vi "ReadAllDataByLabVIEW.vi"() -> ()   [LabVIEW 2020]
panel:
  in  "CreateSupportRequest":bool caption="Create\nSupport Request\n       Textfile"
  out "cSupportRequestText":string
  out "cProductModel":string caption="Product Model"
  out "cLastErrorPhase":string
  out "cLastErrorText":string
  out "clLastFWError":T1
  out "cModulesDisplay":string
  out "error out":errorcluster {"code" format="%9.0d"}
  out "iModuleCount":i32 caption="Modules"
  in  "error in (no error)":errorcluster
  out "cSerialNumber":string caption="Serial Number"
  in  "iDevIdx":i32 caption="Device Index" min=0 max=7 step=1
  in  "iPerformRestart":bool caption="Restart"
  out "cDescriptor":string caption="Descriptor"
  # "Module-by-Module\nSystem Analysis"
  # "System Description\nfor\nSupport Requests"
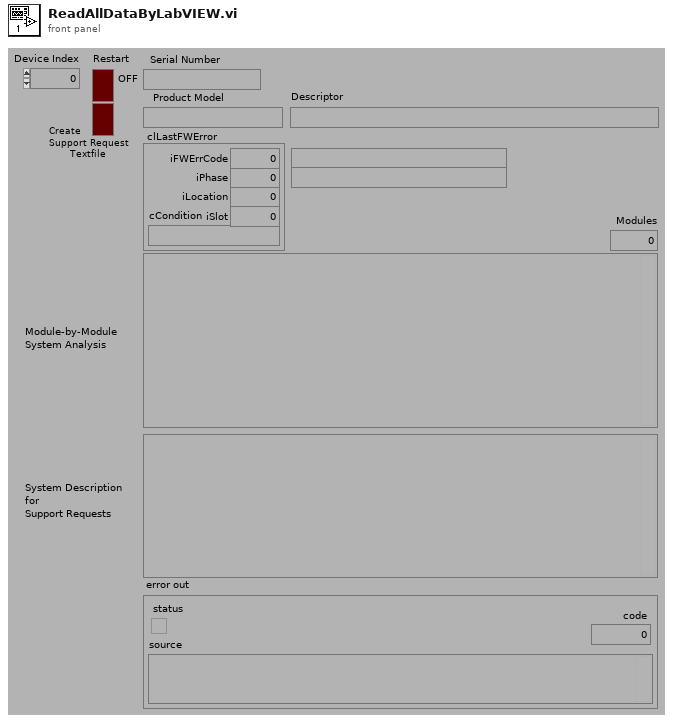
[diagram p1: front panel]
types:
  T1 = cluster{"iFWErrCode":i32, "iPhase":i32, "iLocation":i32, "iSlot":i32, "cCondition":string}
  T2 = cluster{"ErrCode":i32, "Error Text":string, "Phase":i32, "Phase Text":string, "Location":i32, "Slot":i32, "Condition":string}
  T3 = cluster{"SlotId":i32, "IsPrimary":u8, "IsBackPlane":u8, "HasUptimeCounter":u8}
  T4 = cluster{"TBNdxCount":u8, "MaxAmplitude":u16, "MaxSlewRate":u16, "ExpRampEffect":u16, "MinUserValue":u16, "MaxUserValue":u16, "UserResolution":u16}
  T5 = cluster{"TBNdx":u8, "PAPml":u16, "RRPml":u16, "PSPml":u16, "RSPml":u16, "WSPml":u16}
  T6 = cluster{"PumpState":enum8{"BOOST", "ECO"}, "PumpMode":enum8{"static", "dynamic"}}
  T7 = cluster{"Divider":u8, "PreSync":u8, "SyncMask":u8}
  T8 = cluster{"OutEnable":u8, "SyncEnable":u8, "SyncInverse":enum8{"Standard_Sync_Mask", "Inverse_Sync_Mask"}}
  T9 = cluster{"Divider":u16, "PreSync":u8, "SyncMask":u8}
  T10 = cluster{"Freq":i32, "PulseMode":u8, "HeadType":i32}
  T11 = cluster{"MainFreqTrig":string, "MainFreq":i32, "TrigLevelEnabled":u8}[]
  T12 = cluster{"MainFreqTrig":string, "MainFreq":i32, "TrigLevelEnabled":u8}
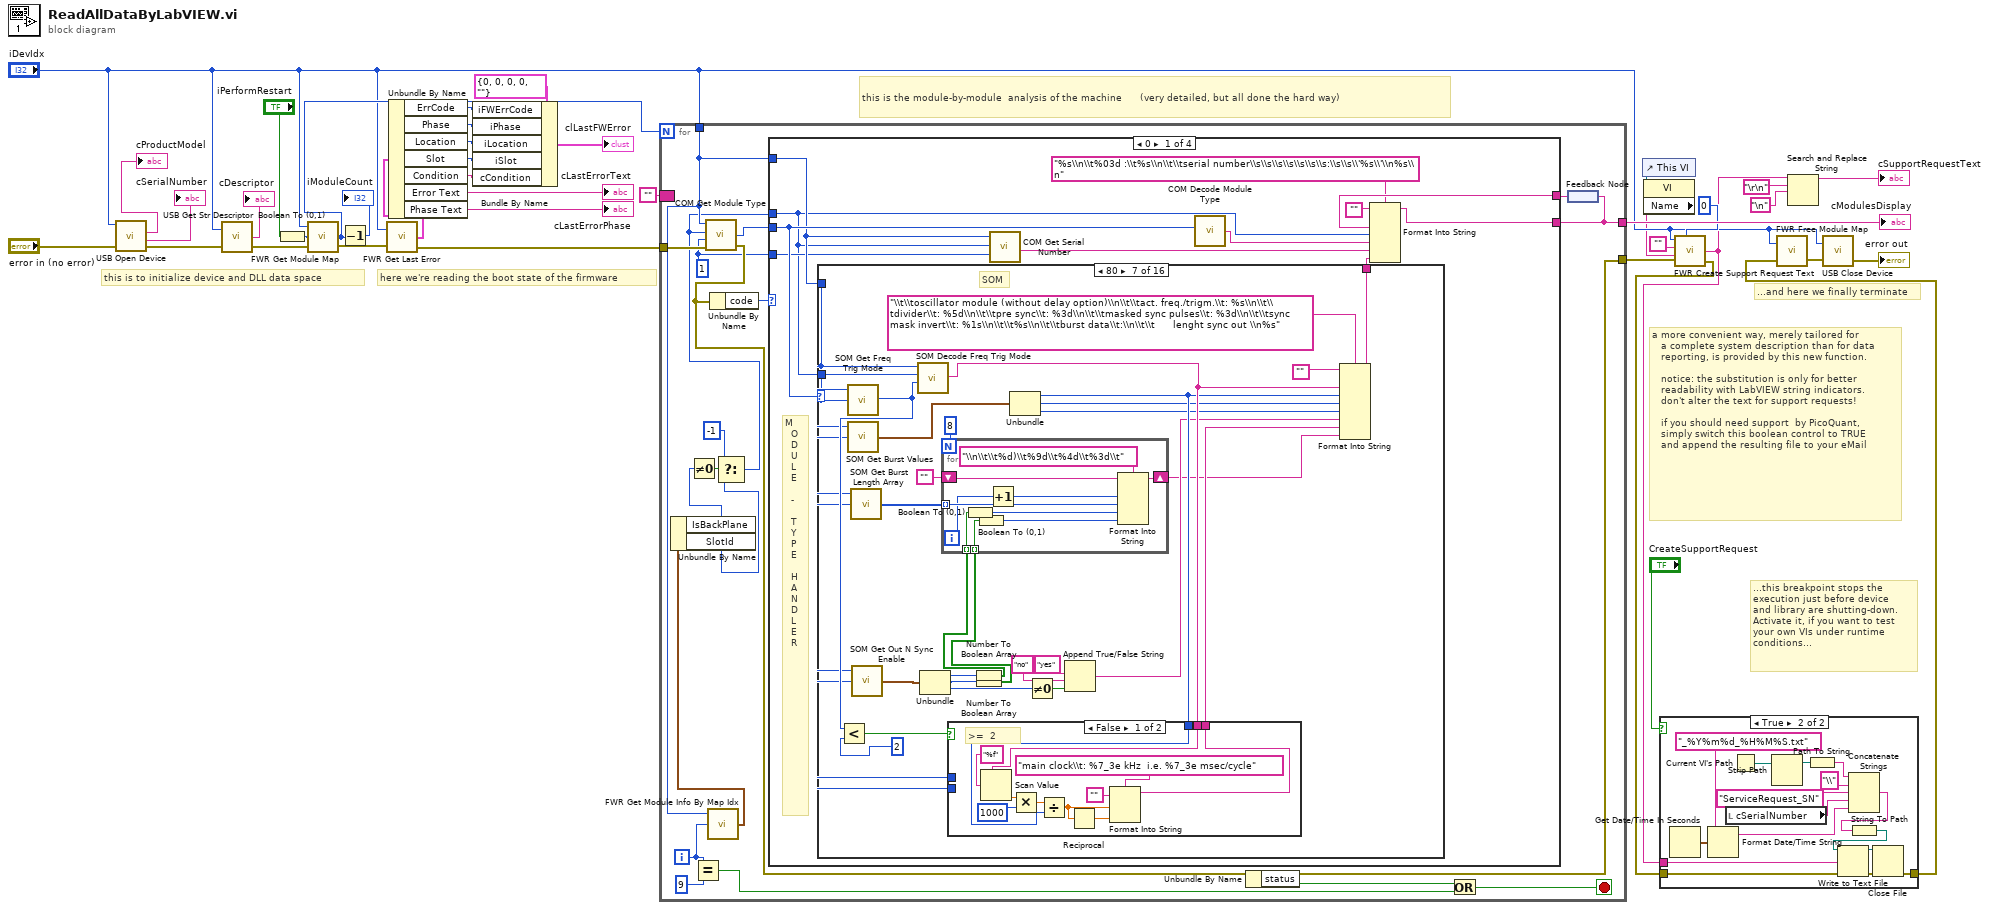
[diagram p0: block diagram]
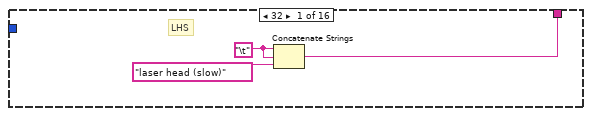
[diagram p3: hidden frame]
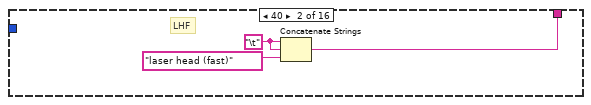
[diagram p4: hidden frame]
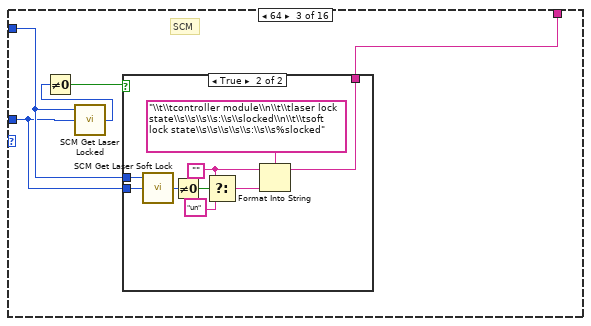
[diagram p5: hidden frame]
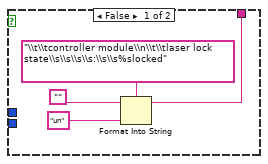
[diagram p6: hidden frame]
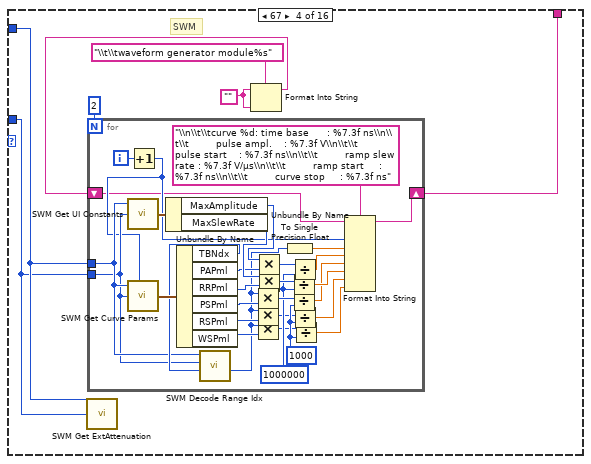
[diagram p7: hidden frame]
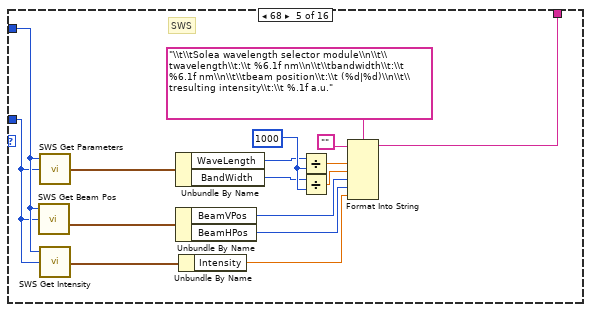
[diagram p8: hidden frame]
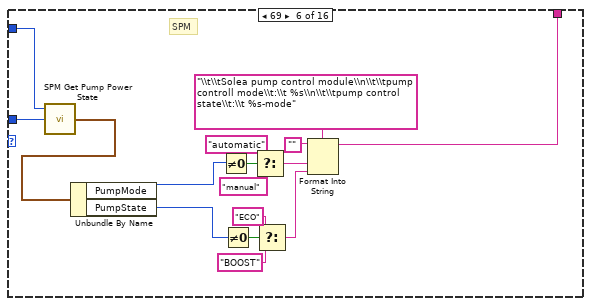
[diagram p9: hidden frame]
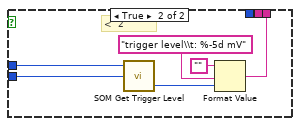
[diagram p10: hidden frame]
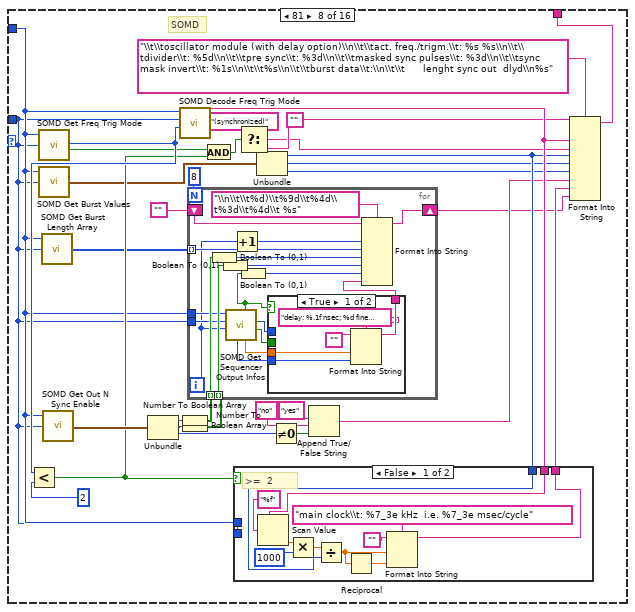
[diagram p11: hidden frame]
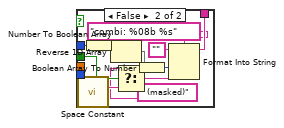
[diagram p12: hidden frame]
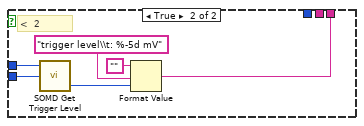
[diagram p13: hidden frame]
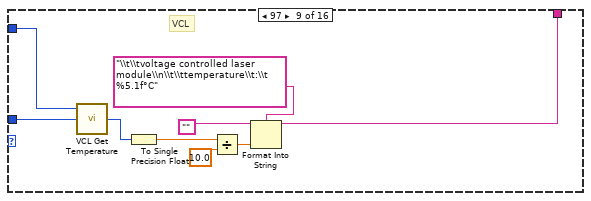
[diagram p14: hidden frame]
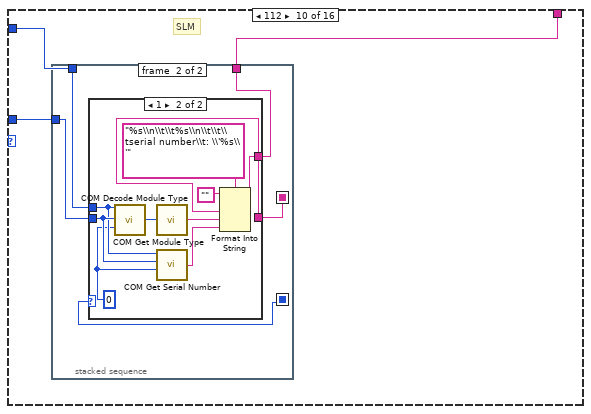
[diagram p15: hidden frame]
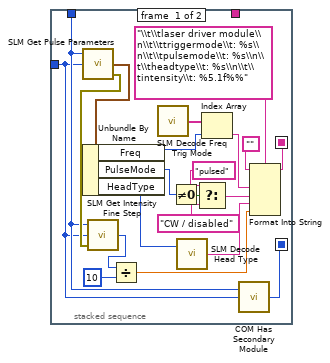
[diagram p16: hidden frame]
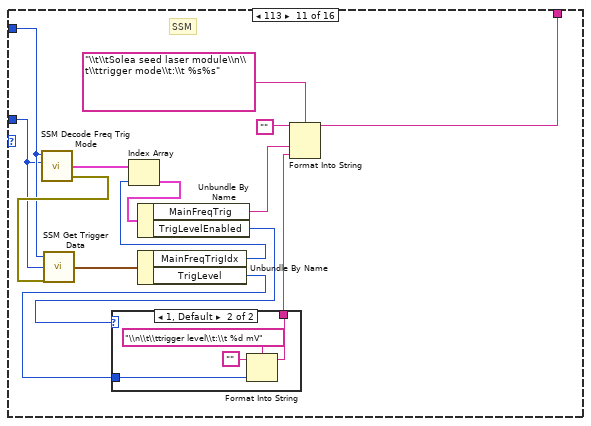
[diagram p18: hidden frame]
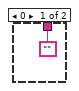
[diagram p19: hidden frame]
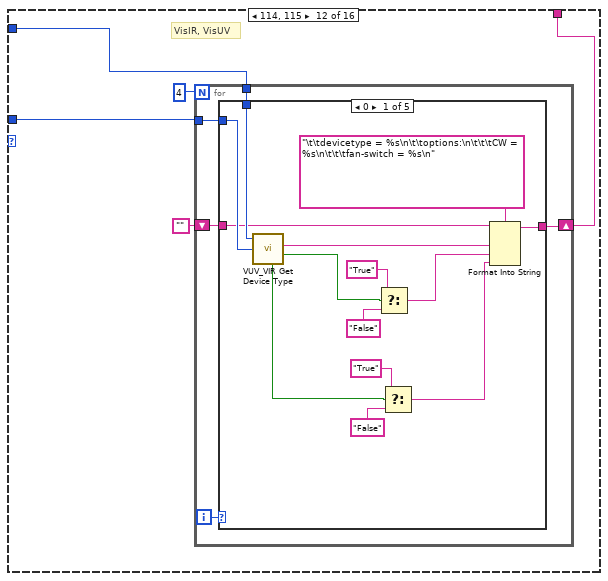
[diagram p20: hidden frame]
diagram:
  # "...this breakpoint stops the\nexecution just before device \nand library are shutting-down. \nActivate it, if you want to test \nyour own VIs under runtime \nconditions..."
  # "here we're reading the boot state of the firmware"
  # "a more convenient way, merely tailored for \n   a complete system description than for data      \n   reporting, is provided by this new function. \n\n   notice: the substitution is only for better  \n   readability with LabVIEW string indicators.\n   don't alter the text for support requests!\n\n   if you should need support  by PicoQuant,\n   simply switch this boolean control to TRUE\n   and append the resulting file to your eMail"
  # "...and here we finally terminate"
  # "this is the module-by-module  analysis of the machine      (very detailed, but all done the hard way)"
  # "this is to initialize device and DLL data space"
  n1 = call "USB Open Device.vi"("error in (no error)"="error in (no error)", "DevIdx"="iDevIdx") -> ("error out"=w36:errorcluster, "SerialNumber"=→"cSerialNumber":string, "ProductModel"=→"cProductModel":string)  [unwired: 2 in, 1 out]
  n2 = call "USB Get Str Descriptor.vi"("DevIdx"="iDevIdx", "error in (no error)"=w36) -> ("Descriptor"=→"cDescriptor":string, "error out"=w37:errorcluster)  [unwired: 1 out]
  n3 = Boolean To (0,1)(Boolean="iPerformRestart") -> (0, 1=w26:i16)
  n4 = call "FWR Get Module Map.vi"("error in (no error)"=w37, "PerformRestart"=w26, "DevIdx"="iDevIdx") -> ("error out"=w34:errorcluster, "ModuleCount"=w14:i32)  [unwired: 1 out]
  n5 = Decrement(x=w14) -> (x-1=→"iModuleCount":i32)
  n6 = call "FWR Get Last Error.vi"("DevIdx"="iDevIdx", "error in (no error)"=w34) -> ("Last Error"=w23:T2, "error out"=w33:errorcluster)  [unwired: 1 out]
  n7 = Unbundle By Name(w23) -> ("ErrCode"=w22:i32, "Phase"=w21:i32, "Location"=w20:i32, "Slot"=w19:i32, "Condition"=w18:string, "Error Text"=→"cLastErrorText":string, "Phase Text"=→"cLastErrorPhase":string)
  n8 = Bundle By Name(cluster=T1 {"iFWErrCode"=0, "iPhase"=0, "iLocation"=0, "iSlot"=0, "cCondition"=""} ("clLastFWError"), "iFWErrCode"=w22, "iPhase"=w21, "iLocation"=w20, "iSlot"=w19, "cCondition"=w18) -> (→"clLastFWError":T1)
  n9 = for {
    N: w14 -> [_]
    tunnel: "iDevIdx" -> [w45]
    tunnel: [w58] -> w29
    tunnel: w33 -> [w53]
    tunnel: [w52] -> w13
    border: "" -> [_]
    i -> [w48]
    stop <- w46 stop-if-true
    w50 = u8 1
    n10 = Equal?(x=w48, y=9) -> (x = y?=w55:bool)
    n11 = call "FWR Get Module Info By Map Idx.vi"("MapIdx"=w48, "DevIdx"=w45) -> ("FWR Module Info"=w47:T3)  [unwired: 1 in, 2 out]
    n12 = Unbundle By Name(w47) -> ("IsBackPlane"=w40:u8, "SlotId"=w42:i32)
    n13 = Not Equal To 0?(x=w40) -> (x != 0?=w44:bool)
    n14 = Select(t=-1, s=w44, f=w42) -> (s? t:f=w41:i32)
    n15 = call "COM Get Module Type.vi"("error in (no error)"=w53, "GetPrimary"=w50, "SlotId"=w41, "DevIdx"=w45) -> ("error out"=w52:errorcluster, "ModuleType"=w49:i32)  [unwired: 1 out]
    n16 = Unbundle By Name(w52) -> ("code"=w54:i32)
    n17 = Unbundle By Name(w52) -> ("status"=w51:bool)
    n18 = Or(x=w51, y=w55) -> (x .or. y?=w46:bool)
    n19 = feedback #1() -> (w57:string)
    n20 = case shown="0" w54 {
      tunnel: [w63 w604 w610 w616] -> w58
      tunnel: w57 -> [w65 w605 w611 w617]
      tunnel: w49 -> [w69 _ _ _]
      tunnel: w45 -> [w68 _ _ _]
      tunnel: w41 -> [w62 w603 w609 w615]
      tunnel: w50 -> [w67 _ _ _]
      frame 0 {
        # "M\n  O\n  D\n  U\n  L\n  E\n\n  -\n\n  T\n  Y\n  P\n  E\n\n  H\n  A\n  N\n  D\n  L\n  E\n  R"
        n21 = case shown="80" w69 {
          tunnel: [w70 w74 w76 w99 w133 w148 w190 w219 w303 w312 w352 w371 w446 w595 w598 "  oops?"] -> w59
          tunnel: w68 -> [_ _ w80 w98 w147 w163 w171 w221 w311 w314 w362 w375 w445 _ _ _]
          tunnel: w62 -> [_ _ w79 w97 w146 w162 w170 w220 w310 w313 w361 w374 w444 _ _ _]
          frame 32 {
            w72 = "\t"
            # "LHS"
            n22 = Concatenate Strings(w72, w72, "laser head (slow)") -> (w70:string)
          }
          frame 40 {
            w75 = "\t"
            # "LHF"
            n23 = Concatenate Strings(w75, w75, "laser head (fast)") -> (w74:string)
          }
          frame 64 {
            # "SCM"
            n24 = call "SCM Get Laser Locked.vi"("SlotId"=w79, "DevIdx"=w80) -> ("LaserLocked"=w78:enum8{"Laser unlocked", "Laser locked"})  [unwired: 1 in, 2 out]
            n25 = Not Equal To 0?(x=w78) -> (x != 0?=w77:bool)
            n26 = case shown="True" w77 {
              tunnel: [w82 w92] -> w76
              tunnel: w80 -> [_ w91]
              tunnel: w79 -> [_ w90]
              frame False {
                n27 = Format Into String(format string="\\t\\tcontroller module\\n\\t\\tlaser lock state\\s\\s\\s\\s:\\s\\s%slocked", initial string="", "un") -> (resulting string=w82:string)  [unwired: 1 in, 1 out]
              }
              frame True {
                w85 = ""
                n28 = call "SCM Get Laser Soft Lock.vi"("SlotId"=w90, "DevIdx"=w91) -> ("SoftLocked"=w87:enum8{"SoftLock off", "SoftLock on"})  [unwired: 1 in, 2 out]
                n29 = Not Equal To 0?(x=w87) -> (x != 0?=w86:bool)
                n30 = Select(t=w85, s=w86, f="un") -> (s? t:f=w89:string)
                n31 = Format Into String(format string="\\t\\tcontroller module\\n\\t\\tlaser lock state\\s\\s\\s\\s:\\s\\slocked\\n\\t\\tsoft lock state\\s\\s\\s\\s\\s:\\s\\s%slocked", initial string=w85, w89) -> (resulting string=w92:string)  [unwired: 1 in, 1 out]
              }
            }
          }
          frame 67 {
            w95 = ""
            # "SWM"
            n32 = call "SWM Get ExtAttenuation.vi"("SlotId"=w97, "DevIdx"=w98) -> ()  [unwired: 1 in, 3 out]
            n33 = Format Into String(format string="\\t\\twaveform generator module%s", initial string=w95, w95) -> (resulting string=w94:string)  [unwired: 1 in, 1 out]
            n34 = for {
              N: 2 -> [_]
              tunnel: w98 -> [w125]
              tunnel: w97 -> [w124]
              shift-right: [w116] -> w99
              shift-left: w94 -> [w115]
              i -> [w131]
              w110 = 1000
              w111 = 1000000
              n35 = call "SWM Get UI Constants.vi"("SlotId"=w124, "DevIdx"=w125) -> ("SWM UI Constants"=w123:T4)  [unwired: 1 in, 2 out]
              n36 = Increment(x=w131) -> (x+1=w118:i32)
              n37 = call "SWM Get Curve Params.vi"("DevIdx"=w125, "CurveIdx"=w118, "SlotId"=w124) -> ("SWM Curve Params"=w130:T5)  [unwired: 2 in, 2 out]
              n38 = Unbundle By Name(w123) -> ("MaxAmplitude"=w121:u16, "MaxSlewRate"=w122:u16)
              n39 = Unbundle By Name(w130) -> ("TBNdx"=w129:u8, "PAPml"=w120:u16, "RRPml"=w119:u16, "PSPml"=w128:u16, "RSPml"=w127:u16, "WSPml"=w126:u16)
              n40 = call "SWM Decode Range Idx.vi"("RangeIdx"=w129, "SlotId"=w124, "DevIdx"=w125) -> ("UpperLimit"=w101:i32)  [unwired: 2 in, 2 out]
              n41 = Multiply(x=w101, y=w128) -> (x*y=w112:u32)
              n42 = Multiply(x=w101, y=w127) -> (x*y=w109:u32)
              n43 = Multiply(x=w101, y=w126) -> (x*y=w108:u32)
              n44 = Multiply(x=w121, y=w120) -> (x*y=w114:u32)
              n45 = Multiply(x=w122, y=w119) -> (x*y=w113:u32)
              n46 = To Single Precision Float(number=w101) -> (single precision float=w102:sgl)
              n47 = Divide(x=w113, y=w111) -> (x/y=w105:sgl)
              n48 = Divide(x=w112, y=w110) -> (x/y=w104:sgl)
              n49 = Divide(x=w114, y=w111) -> (x/y=w103:sgl)
              n50 = Divide(x=w109, y=w110) -> (x/y=w106:sgl)
              n51 = Divide(x=w108, y=w110) -> (x/y=w107:sgl)
              n52 = Format Into String(format string="\\n\\t\\tcurve %d: time base      : %7.3f ns\\n\\t\\t         pulse ampl.    : %7.3f V\\n\\t\\t         pulse start    : %7.3f ns\\n\\t\\t         ramp slew rate : %7.3f V/µs\\n\\t\\t         ramp start     : %7.3f ns\\n\\t\\t         curve stop     : %7.3f ns", initial string=w115, w118, w102, w103, w104, w105, w106, w107) -> (resulting string=w116:string)  [unwired: 1 in, 1 out]
            }
          }
          frame 68 {
            w144 = 1000
            # "SWS"
            n53 = call "SWS Get Beam Pos.vi"("SlotId"=w146, "DevIdx"=w147) -> ("SWS Beam Pos"=w138:cluster{"BeamVPos":i16, "BeamHPos":i16})  [unwired: 1 in, 2 out]
            n54 = call "SWS Get Parameters.vi"("SlotId"=w146, "DevIdx"=w147) -> ("SWS Parameters"=w145:cluster{"WaveLength":u32, "BandWidth":u32})  [unwired: 1 in, 2 out]
            n55 = call "SWS Get Intensity.vi"("SlotId"=w146, "DevIdx"=w147) -> ("SWS Intensity"=w137:cluster{"IntensityRaw":u32, "Intensity":sgl})  [unwired: 1 in, 2 out]
            n56 = Unbundle By Name(w145) -> ("WaveLength"=w142:u32, "BandWidth"=w143:u32)
            n57 = Unbundle By Name(w138) -> ("BeamVPos"=w136:i16, "BeamHPos"=w135:i16)
            n58 = Unbundle By Name(w137) -> ("Intensity"=w134:sgl)
            n59 = Divide(x=w142, y=w144) -> (x/y=w140:sgl)
            n60 = Divide(x=w143, y=w144) -> (x/y=w139:sgl)
            n61 = Format Into String(format string="\\t\\tSolea wavelength selector module\\n\\t\\twavelength\\t:\\t %6.1f nm\\n\\t\\tbandwidth\\t:\\t %6.1f nm\\n\\t\\tbeam position\\t:\\t (%d|%d)\\n\\t\\tresulting intensity\\t:\\t %.1f a.u.", initial string="", w140, w139, w136, w135, w134) -> (resulting string=w133:string)  [unwired: 1 in, 1 out]
          }
          frame 69 {
            # "SPM"
            n62 = call "SPM Get Pump Power State.vi"("SlotId"=w162, "DevIdx"=w163) -> ("Pump Power State"=w161:T6)  [unwired: 1 in, 2 out]
            n63 = Unbundle By Name(w161) -> ("PumpMode"=w151:enum8{"static", "dynamic"}, "PumpState"=w150:enum8{"BOOST", "ECO"})
            n64 = Not Equal To 0?(x=w151) -> (x != 0?=w159:bool)
            n65 = Not Equal To 0?(x=w150) -> (x != 0?=w155:bool)
            n66 = Select(t="automatic", s=w159, f="manual") -> (s? t:f=w160:string)
            n67 = Select(t="ECO", s=w155, f="BOOST") -> (s? t:f=w152:string)
            n68 = Format Into String(format string="\\t\\tSolea pump control module\\n\\t\\tpump controll mode\\t:\\t %s\\n\\t\\tpump control state\\t:\\t %s-mode", initial string="", w160, w152) -> (resulting string=w148:string)  [unwired: 1 in, 1 out]
          }
          frame 80 {
            # "SOM"
            n69 = call "SOM Get Freq Trig Mode.vi"("SlotId"=w170, "DevIdx"=w171) -> ("FreqTrigMode"=w184:i32)  [unwired: 1 in, 2 out]
            n70 = Less?(x=w184, y=2) -> (x < y?=w183:bool)
            n71 = call "SOM Get Burst Values.vi"("SlotId"=w170, "DevIdx"=w171) -> ("SOM Burst Values"=w182:T7)  [unwired: 1 in, 2 out]
            n72 = call "SOM Get Burst Length Array.vi"("SlotId"=w170, "DevIdx"=w171) -> ("SOM Burst Length Array"=w180:i32[])  [unwired: 1 in, 2 out]
            n73 = call "SOM Get Out N Sync Enable.vi"("SlotId"=w170, "DevIdx"=w171) -> ("SOM Out N Sync Enable"=w187:T8)  [unwired: 1 in, 2 out]
            n74 = call "SOM Decode Freq Trig Mode.vi"("FreqTrigMode"=w184, "SlotId"=w170, "DevIdx"=w171) -> ("FreqTrigMode"=w188:string)  [unwired: 1 in, 2 out]
            n75 = Unbundle(w187) -> ("OutEnable"=w175:u8, "SyncEnable"=w176:u8, "SyncInverse"=w186:enum8{"Standard_Sync_Mask", "Inverse_Sync_Mask"})
            n76 = Number To Boolean Array(number=w175) -> (Boolean array=w174:bool[])
            n77 = Number To Boolean Array(number=w176) -> (Boolean array=w173:bool[])
            n78 = for {
              N: 8 -> [_]
              tunnel: w180 -> [w201] mode=indexing
              shift-right: [w198] -> w164
              shift-left: "" -> [w197]
              tunnel: w174 -> [w194] mode=indexing
              tunnel: w173 -> [w193] mode=indexing
              i -> [w192]
              n79 = Boolean To (0,1)(Boolean=w194) -> (0, 1=w196:i16)
              n80 = Boolean To (0,1)(Boolean=w193) -> (0, 1=w195:i16)
              n81 = Increment(x=w192) -> (x+1=w200:i32)
              n82 = Format Into String(format string="\\n\\t\\t%d)\\t%9d\\t%4d\\t%3d\\t", initial string=w197, w200, w201, w196, w195) -> (resulting string=w198:string)  [unwired: 1 in, 1 out]
            }
            n83 = Unbundle(w182) -> ("Divider"=w169:u8, "PreSync"=w168:u8, "SyncMask"=w167:u8)
            n84 = case shown="False" w183 {
              tunnel: w171 -> [_ w218]
              tunnel: w170 -> [_ w217]
              tunnel: [w211 w213] -> w165
              tunnel: w188 -> [w202 _]
              tunnel: w169 -> [w203 _]
              frame False {
                # ">=  2"
                n85 = Scan Value(string=w202, format string="%f") -> (value=w208:dbl)  [unwired: 1 in, 1 out]
                n86 = Multiply(x=w208, y=1000) -> (x*y=w206:dbl)
                n87 = Divide(x=w206, y=w203) -> (x/y=w205:dbl)
                n88 = Reciprocal(x=w205) -> (1/x=w204:dbl)
                n89 = Format Into String(format string="main clock\\t: %7_3e kHz  i.e. %7_3e msec/cycle", initial string="", w205, w204) -> (resulting string=w211:string)  [unwired: 1 in, 1 out]
              }
              frame True {
                # "<  2"
                n90 = call "SOM Get Trigger Level.vi"("SlotId"=w217, "DevIdx"=w218) -> ("MilliVolt"=w216:i32)  [unwired: 1 in, 2 out]
                n91 = Format Value(string ("")="", format string="trigger level\\t: %-5d mV", value (0)=w216) -> (output string=w213:string)
              }
            }
            n92 = Not Equal To 0?(x=w186) -> (x != 0?=w179:bool)
            n93 = Append True/False String(1:w179, 2:"no" ("false string"), 3:"yes" ("true string")) -> (0:w166:string)  [unwired: 1 in]
            n94 = Format Into String(format string="\\t\\toscillator module (without delay option)\\n\\t\\tact. freq./trigm.\\t: %s\\n\\t\\tdivider\\t: %5d\\n\\t\\tpre sync\\t: %3d\\n\\t\\tmasked sync pulses\\t: %3d\\n\\t\\tsync mask invert\\t: %1s\\n\\t\\t%s\\n\\t\\tburst data\\t:\\n\\t\\t      lenght sync out \\n%s", initial string="", w188, w169, w168, w167, w166, w165, w164) -> (resulting string=w190:string)  [unwired: 1 in, 1 out]
          }
          frame 81 {
            w245 = ""
            # "SOMD"
            n95 = call "SOMD Get Freq Trig Mode.vi"("DevIdx"=w221, "SlotId"=w220) -> ("FreqTrigMode"=w243:i32, "Synchronize"=w241:bool)  [unwired: 1 in, 2 out]
            n96 = Less?(x=w243, y=2) -> (x < y?=w240:bool)
            n97 = call "SOMD Get Burst Values.vi"("SlotId"=w220, "DevIdx"=w221) -> ("SOMD Burst Values"=w239:T9)  [unwired: 1 in, 2 out]
            n98 = call "SOMD Get Burst Length Array.vi"("SlotId"=w220, "DevIdx"=w221) -> ("SOMD Burst Length Array"=w235:i32[])  [unwired: 1 in, 2 out]
            n99 = call "SOMD Get Out N Sync Enable.vi"("SlotId"=w220, "DevIdx"=w221) -> ("SOMD Out N Sync Enable"=w247:T8)  [unwired: 1 in, 2 out]
            n100 = Unbundle(w247) -> ("OutEnable"=w226:u8, "SyncEnable"=w227:u8, "SyncInverse"=w246:enum8{"Standard_Sync_Mask", "Inverse_Sync_Mask"})
            n101 = call "SOMD Decode Freq Trig Mode.vi"("FreqTrigMode"=w243, "SlotId"=w220, "DevIdx"=w221) -> ("FreqTrigMode"=w248:string)  [unwired: 1 in, 2 out]
            n102 = Number To Boolean Array(number=w226) -> (Boolean array=w225:bool[])
            n103 = Number To Boolean Array(number=w227) -> (Boolean array=w224:bool[])
            n104 = for {
              N: 8 -> [_]
              tunnel: w235 -> [w269] mode=indexing
              shift-right: [w266] -> w222
              shift-left: "" -> [w265]
              tunnel: w225 -> [w262] mode=indexing
              tunnel: w224 -> [w261] mode=indexing
              tunnel: w221 -> [w260]
              tunnel: w220 -> [w259]
              i -> [w258]
              n105 = Boolean To (0,1)(Boolean=w262) -> (0, 1=w264:i16)
              n106 = Boolean To (0,1)(Boolean=w261) -> (0, 1=w263:i16)
              n107 = call "SOMD Get Sequencer Output Infos.vi"("SeqOutputIdx"=w258, "SlotId"=w259, "DevIdx"=w260) -> ("Masked Combi"=w251:bool, "bOutputCombi"=w252:u8, "Coarse Delay"=w255:dbl, "Delayed"=w256:bool, "Fine Delay"=w254:u8)  [unwired: 1 in, 3 out]
              n108 = Increment(x=w258) -> (x+1=w268:i32)
              n109 = Boolean To (0,1)(Boolean=w256) -> (0, 1=w257:i16)
              n110 = case shown="True" w256 {
                tunnel: w255 -> [w274 _]
                tunnel: w254 -> [w273 _]
                tunnel: [w271 w284] -> w253
                tunnel: w252 -> [_ w282]
                tunnel: w251 -> [_ w278]
                frame True {
                  n111 = Format Into String(format string="delay: %.1f nsec; %d fine steps", initial string="", w274, w273) -> (resulting string=w271:string)  [unwired: 1 in, 1 out]
                }
                frame False {
                  n112 = call <vilib>:"Space Constant.vi"() -> ("String"=w277:string)
                  n113 = Number To Boolean Array(number=w282) -> (Boolean array=w281:bool[])
                  n114 = Reverse 1D Array(array=w281) -> (reversed array=w280:bool[])
                  n115 = Select(t=" (masked)", s=w278, f=w277) -> (s? t:f=w275:string)
                  n116 = Boolean Array To Number(Boolean array=w280) -> (number=w279:u8)
                  n117 = Format Into String(format string="combi: %08b %s", initial string="", w279, w275) -> (resulting string=w284:string)  [unwired: 1 in, 1 out]
                }
              }
              n118 = Format Into String(format string="\\n\\t\\t%d)\\t%9d\\t%4d\\t%3d\\t%4d\\t %s", initial string=w265, w268, w269, w264, w263, w257, w253) -> (resulting string=w266:string)  [unwired: 1 in, 1 out]
            }
            n119 = And(x=w241, y=w240) -> (x .and. y?=w242:bool)
            n120 = Select(t="(synchronized)", s=w242, f=w245) -> (s? t:f=w238:string)
            n121 = Unbundle(w239) -> ("Divider"=w237:u16, "PreSync"=w231:u8, "SyncMask"=w230:u8)
            n122 = case shown="False" w240 {
              tunnel: w221 -> [_ w302]
              tunnel: w220 -> [_ w301]
              tunnel: [w295 w297] -> w228
              tunnel: w248 -> [w286 _]
              tunnel: w237 -> [w287 _]
              frame False {
                # ">=  2"
                n123 = Scan Value(string=w286, format string="%f") -> (value=w292:dbl)  [unwired: 1 in, 1 out]
                n124 = Multiply(x=w292, y=1000) -> (x*y=w290:dbl)
                n125 = Divide(x=w290, y=w287) -> (x/y=w289:dbl)
                n126 = Reciprocal(x=w289) -> (1/x=w288:dbl)
                n127 = Format Into String(format string="main clock\\t: %7_3e kHz  i.e. %7_3e msec/cycle", initial string="", w289, w288) -> (resulting string=w295:string)  [unwired: 1 in, 1 out]
              }
              frame True {
                # "<  2"
                n128 = call "SOMD Get Trigger Level.vi"("SlotId"=w301, "DevIdx"=w302) -> ("MilliVolt"=w300:i32)  [unwired: 1 in, 2 out]
                n129 = Format Value(string ("")="", format string="trigger level\\t: %-5d mV", value (0)=w300) -> (output string=w297:string)
              }
            }
            n130 = Not Equal To 0?(x=w246) -> (x != 0?=w234:bool)
            n131 = Append True/False String(1:w234, 2:"no" ("false string"), 3:"yes" ("true string")) -> (0:w229:string)  [unwired: 1 in]
            n132 = Format Into String(format string="\\t\\toscillator module (with delay option)\\n\\t\\tact. freq./trigm.\\t: %s %s\\n\\t\\tdivider\\t: %5d\\n\\t\\tpre sync\\t: %3d\\n\\t\\tmasked sync pulses\\t: %3d\\n\\t\\tsync mask invert\\t: %1s\\n\\t\\t%s\\n\\t\\tburst data\\t:\\n\\t\\t      lenght sync out  dlyd\\n%s", initial string=w245, w248, w238, w237, w231, w230, w229, w228, w222) -> (resulting string=w219:string)  [unwired: 1 in, 1 out]
          }
          frame 97 {
            # "VCL"
            n133 = call "VCL Get Temperature.vi"("SlotId"=w310, "DevIdx"=w311) -> ("Temperature / 0.1 °C"=w304:i32)  [unwired: 1 in, 2 out]
            n134 = To Single Precision Float(number=w304) -> (single precision float=w305:sgl)
            n135 = Divide(x=w305, y=sgl 10.0) -> (x/y=w306:sgl)
            n136 = Format Into String(format string="\\t\\tvoltage controlled laser module\\n\\t\\ttemperature\\t:\\t %5.1f°C", initial string="", w306) -> (resulting string=w303:string)  [unwired: 1 in, 1 out]
          }
          frame 112 {
            # "SLM"
            n137 = stacked-sequence {
              seq-local: [w330 _] -> [_ w339]
              seq-local: [w315 _] -> [_ w336]
              tunnel: w314 -> [w328 w338]
              tunnel: w313 -> [w327 w337]
              tunnel: [_ w340] -> w312
              frame #0 {
                n138 = call "SLM Get Pulse Parameters.vi"("SlotId"=w327, "DevIdx"=w328) -> ("error out"=w329:errorcluster, "SLM Pulse Parameters"=w323:T10)  [unwired: 1 in, 1 out]
                n139 = Unbundle By Name(w323) -> ("Freq"=w322:i32, "PulseMode"=w316:u8, "HeadType"=w318:i32)
                n140 = call "SLM Get Intensity Fine Step.vi"("error in (no error)"=w329, "SlotId"=w327, "DevIdx"=w328) -> ("Intensity"=w326:u16)  [unwired: 2 out]
                n141 = Divide(x=w326, y=10) -> (x/y=w324:dbl)
                n142 = call "SLM Decode Freq Trig Mode.vi"() -> ("FreqTrigMode"=w320:string[])  [unwired: 2 in, 2 out]
                n143 = Not Equal To 0?(x=w316) -> (x != 0?=w317:bool)
                n144 = call "SLM Decode Head Type.vi"("HeadType"=w318) -> ("HeadType"=w334:string)  [unwired: 1 in, 2 out]
                n145 = Select(t="pulsed", s=w317, f="CW / disabled") -> (s? t:f=w332:string)
                n146 = Index Array(array=w320, index=w322) -> (element=w321:string)
                n147 = call "COM Has Secondary Module.vi"("SlotId"=w327, "DevIdx"=w328) -> ("HasSecondary"=w315:i32)  [unwired: 1 in, 2 out]
                n148 = Format Into String(format string="\\t\\tlaser driver module\\n\\t\\ttriggermode\\t: %s\\n\\t\\tpulsemode\\t: %s\\n\\t\\theadtype\\t: %s\\n\\t\\tintensity\\t: %5.1f%%", initial string="", w321, w332, w334, w324) -> (resulting string=w330:string)  [unwired: 1 in, 1 out]
              }
              frame #1 {
                n149 = case shown="1" w336 {
                  tunnel: [w341 w351] -> w340
                  tunnel: w339 -> [w341 w343]
                  tunnel: w338 -> [_ w345]
                  tunnel: w337 -> [_ w346]
                  frame 0, Default {
                  }
                  frame 1 {
                    w342 = u8 0
                    n150 = call "COM Get Module Type.vi"("GetPrimary"=w342, "SlotId"=w346, "DevIdx"=w345) -> ("function return"=w347:i32)  [unwired: 1 in, 2 out]
                    n151 = call "COM Decode Module Type.vi"("ModuleType"=w347) -> ("ModulType"=w349:string)  [unwired: 1 in, 2 out]
                    n152 = call "COM Get Serial Number.vi"("GetPrimary"=w342, "SlotId"=w346, "DevIdx"=w345) -> ("SerialNumber"=w350:string)  [unwired: 1 in, 2 out]
                    n153 = Format Into String(format string="%s\\n\\t\\t%s\\n\\t\\t\\tserial number\\t: \\'%s\\'", initial string="", w343, w349, w350) -> (resulting string=w351:string)  [unwired: 1 in, 1 out]
                  }
                }
              }
            }
          }
          frame 113 {
            # "SSM"
            n154 = call "SSM Decode Freq Trig Mode.vi"("DevIdx"=w362, "SlotId"=w361) -> ("SSM Trigger Mode"=w360:T11, "error out"=w363:errorcluster)  [unwired: 3 in, 1 out]
            n155 = call "SSM Get Trigger Data.vi"("error in (no error)"=w363, "SlotId"=w361, "DevIdx"=w362) -> ("SSM Trigger Data"=w365:cluster{"MainFreqTrigIdx":i32, "TrigLevel":i32})  [unwired: 2 out]
            n156 = Unbundle By Name(w365) -> ("MainFreqTrigIdx"=w359:i32, "TrigLevel"=w353:i32)
            n157 = Index Array(array=w360, index=w359) -> (element=w358:T12)
            n158 = Unbundle By Name(w358) -> ("MainFreqTrig"=w356:string, "TrigLevelEnabled"=w355:u8)
            n159 = case shown="1, Default" w355 {
              tunnel: ["" w367] -> w354
              tunnel: w353 -> [_ w368]
              frame 0 {
              }
              frame 1, Default {
                n160 = Format Into String(format string="\\n\\t\\ttrigger level\\t:\\t %d mV", initial string="", w368) -> (resulting string=w367:string)  [unwired: 1 in, 1 out]
              }
            }
            n161 = Format Into String(format string="\\t\\tSolea seed laser module\\n\\t\\ttrigger mode\\t:\\t %s%s", initial string="", w356, w354) -> (resulting string=w352:string)  [unwired: 1 in, 1 out]
          }
          frame 114, 115 {
            # "VisIR, VisUV"
            n162 = for {
              N: 4 -> [_]
              tunnel: w375 -> [w380]
              tunnel: w374 -> [w379]
              shift-right: [w378] -> w371
              shift-left: "" -> [w376]
              i -> [w377]
              n163 = case shown="0" w377 {
                tunnel: w380 -> [w394 w405 w433 w442 _]
                tunnel: w379 -> [w393 w404 w432 w441 _]
                tunnel: [w390 w409 w430 w439 w443] -> w378
                tunnel: w376 -> [w383 w408 w429 w438 w443]
                frame 0 {
                  n164 = call "VUV_VIR Get Device Type.vi"("DevIdx"=w394, "SlotId"=w393) -> ("DeviceType"=w392:string, "OptCW"=w382:bool, "OptFanSwitch"=w381:bool)  [unwired: 1 in, 2 out]
                  n165 = Select(t="True", s=w382, f="False") -> (s? t:f=w387:string)
                  n166 = Select(t="True", s=w381, f="False") -> (s? t:f=w384:string)
                  n167 = Format Into String(format string="\t\tdevicetype = %s\n\t\toptions:\n\t\t\tCW = %s\n\t\t\tfan-switch = %s\n", initial string=w383, w392, w387, w384) -> (resulting string=w390:string)  [unwired: 1 in, 1 out]
                }
                frame 1 {
                  n168 = call "VUV_VIR Get Trigger Data.vi"("DevIdx"=w405, "SlotId"=w404) -> ("MainTrigSrcIdx"=w403:i32, "MainFreqDivIdx"=w399:i32, "TrigLevel"=w395:i32)  [unwired: 1 in, 2 out]
                  n169 = call "VUV_VIR Decode FreqTrig Mode.vi"("DevIdx"=w405, "SlotId"=w404, "MainTrigSrcIdx"=w403, "MainFreqDivIdx"=w399) -> ("MainFreq"=w398:i32, "TrigDividerEnabled"=w402:bool, "TrigLevelEnabled"=w396:bool)  [unwired: 6 in, 3 out]
                  n170 = call "VUV_VIR Decode FreqTrig Mode.vi"("DevIdx"=w405, "SlotId"=w404, "MainTrigSrcIdx"=w403, "MainFreqDivIdx"=-1) -> ("MainFreqTrig"=w406:string)  [unwired: 6 in, 5 out]
                  n171 = Greater Than 0?(x=w398) -> (x > 0?=w401:bool)
                  n172 = And(x=w401, y=w402) -> (x .and. y?=w400:bool)
                  n173 = case shown="False" w400 {
                    tunnel: w399 -> [_ w423]
                    tunnel: w398 -> [_ w420]
                    tunnel: [w412 w419] -> w397
                    tunnel: w396 -> [w413 _]
                    tunnel: w395 -> [w411 _]
                    frame False {
                      n174 = case shown="True" w413 {
                        tunnel: [_ w417] -> w412
                        tunnel: w411 -> [_ w416]
                        frame False {
                        }
                        frame True {
                          n175 = Multiply(x=w416, y=0.001) -> (x*y=w414:dbl)
                          n176 = Format Into String(format string="\t\ttrigger level = %.3f V\n", w414) -> (resulting string=w417:string)  [unwired: 2 in, 1 out]
                        }
                      }
                    }
                    frame True {
                      n177 = Scale By Power Of 2(n=w423, x=1.0) -> (x*2^n=w422:dbl)
                      n178 = To Long Integer(number=w422) -> (32bit integer=w421:i32)
                      n179 = Format Into String(format string="\t\tdivider = 2^%d = %d\n\t\tfrequency = %d Hz\n", w423, w421, w420) -> (resulting string=w419:string)  [unwired: 2 in, 1 out]
                    }
                  }
                  n180 = Format Into String(format string="\t\ttrigger source = %s\n%s", initial string=w408, w406, w397) -> (resulting string=w409:string)  [unwired: 1 in, 1 out]
                }
                frame 2 {
                  n181 = call "VUV_VIR Get Intensity.vi"("SlotId"=w432, "DevIdx"=w433) -> ("Intensity"=w428:i32)  [unwired: 1 in, 2 out]
                  n182 = Multiply(x=w428, y=0.1) -> (x*y=w426:dbl)
                  n183 = Format Into String(format string="\t\tintensity = %.1f \\%\n", initial string=w429, w426) -> (resulting string=w430:string)  [unwired: 1 in, 1 out]
                }
                frame 3 {
                  n184 = call "VUV_VIR Get Fan.vi"("SlotId"=w441, "DevIdx"=w442) -> ("FanRunning"=w437:bool)  [unwired: 1 in, 2 out]
                  n185 = Select(t="True", s=w437, f="False") -> (s? t:f=w434:string)
                  n186 = Format Into String(format string="\t\tfan running = %s\n", initial string=w438, w434) -> (resulting string=w439:string)  [unwired: 1 in, 1 out]
                }
                frame Default {
                }
              }
            }
          }
          frame 116 {
            # "Prima, Quader"
            n187 = for {
              N: 5 -> [_]
              tunnel: w445 -> [w453]
              tunnel: w444 -> [w452]
              shift-right: [w451] -> w446
              shift-left: "" -> [w449]
              i -> [w450]
              n188 = case shown="4" w450 {
                tunnel: w453 -> [w457 w482 w510 w557 w573 _]
                tunnel: w452 -> [w454 w487 w509 w556 w572 _]
                tunnel: [w469 w489 w537 w560 w589 w594] -> w451
                tunnel: w449 -> [w468 w490 w538 w559 w588 w594]
                frame 0 {
                  n189 = call "PRI Get Device Info.vi"("DevIdx"=w457, "SlotId"=w454) -> ("WL_Count"=w466:i32, "DeviceType"=w465:string, "FW_Version"=w467:string)  [unwired: 1 in, 3 out]
                  n190 = call "PRI Get Wavelengths List.vi"("SlotId"=w454, "DevIdx"=w457) -> ("Wavelengths"=w458:i32[], "ListLen"=w463:i32)  [unwired: 2 in, 2 out]
                  n191 = call "PRI Get Wavelength Index.vi"("SlotId"=w454, "DevIdx"=w457) -> ("Wavelength_Idx"=w456:i32)  [unwired: 1 in, 2 out]
                  n192 = for {
                    N: w463 -> [_]
                    tunnel: w458 -> [w476]
                    shift-right: [w474] -> w461
                    shift-left: "" -> [w473]
                    i -> [w471]
                    n193 = Index Array(array=w476, index=w471) -> (element=w472:i32)
                    n194 = Format Into String(format string="\\t\\t\\s\\swavelength\\s[%d]\\s\\s\\s\\s=\\s\\s%dnm\\n", initial string=w473, w471, w472) -> (resulting string=w474:string)  [unwired: 1 in, 1 out]
                  }
                  n195 = call <vilib>:"Trim Whitespace.vi"("string"=w465) -> ("trimmed string"=w464:string)  [unwired: 1 in]
                  n196 = Index Array(array=w458, index=w456) -> (element=w455:i32)
                  n197 = Format Into String(format string="\\t\\tcur.\\swavelength\\s\\s\\s\\s\\s=\\s\\s%dnm;\\s\\s\\s\\s\\s\\s\\s\\s\\s\\s\\s\\sWL-Idx=%d\\n\\n", w455, w456) -> (resulting string=w460:string)  [unwired: 2 in, 1 out]
                  n198 = Format Into String(format string="\t\tdevicetype          =  '%s'\n\t\tfirmware version    =  %s\n\t\t\n\t\twavelengths count   =  %d\n%s%s", initial string=w468, w464, w467, w466, w461, w460) -> (resulting string=w469:string)  [unwired: 1 in, 1 out]
                }
                frame 1 {
                  n199 = call "PRI Get Operation Modes List.vi"("SlotId"=w487, "DevIdx"=w482) -> ("OpModes_List"=w483:string[], "ListLen"=w484:i32)  [unwired: 2 in, 2 out]
                  n200 = call "PRI Get Operation Mode.vi"("SlotId"=w487, "DevIdx"=w482) -> ("OpMode_Idx"=w478:i32)  [unwired: 1 in, 2 out]
                  n201 = for {
                    N: w484 -> [_]
                    shift-right: [w497] -> w486
                    shift-left: "" -> [w496]
                    tunnel: w483 -> [w493] mode=indexing
                    i -> [w494]
                    n202 = call <vilib>:"Trim Whitespace.vi"("string"=w493) -> ("trimmed string"=w492:string)  [unwired: 1 in]
                    n203 = Format Into String(format string="\\t\\t\\s\\soper. mode [%d]\\s\\s\\s\\s=\\s\\s'%s'\\n", initial string=w496, w494, w492) -> (resulting string=w497:string)  [unwired: 1 in, 1 out]
                  }
                  n204 = call "PRI Decode Operation Mode.vi"("OpMode_Idx"=w478, "SlotId"=w487, "DevIdx"=w482) -> ("OpMode"=w488:string)  [unwired: 1 in, 2 out]
                  n205 = call <vilib>:"Trim Whitespace.vi"("string"=w488) -> ("trimmed string"=w479:string)  [unwired: 1 in]
                  n206 = String Length(string=w479) -> (length=w481:i32)
                  n207 = String Subset(string="';             ", offset (0)=w481) -> (substring=w477:string)  [unwired: 1 in]
                  n208 = Format Into String(format string="\t\toperation modes     =  %d\n%s\t\tcur. oper. mode     =  '%s';%sOM-Idx=%d\n\n", initial string=w490, w484, w486, w479, w477, w478) -> (resulting string=w489:string)  [unwired: 1 in, 1 out]
                }
                frame 2 {
                  w504 = 1000
                  n209 = call "PRI Get Trigger Source.vi"("SlotId"=w509, "DevIdx"=w510) -> ("TrigSrc_Idx"=w507:i32)  [unwired: 1 in, 2 out]
                  n210 = call "PRI Get Trigger Sources Lists.vi"("SlotId"=w509, "DevIdx"=w510) -> ("TrigSrcs_List"=w531:string[], "ListLen"=w532:i32)  [unwired: 2 in, 4 out]
                  n211 = call "PRI Get Trigger Level Limits.vi"("SlotId"=w509, "DevIdx"=w510) -> ("MaxLevel"=w502:i32, "MinLevel"=w503:i32)  [unwired: 2 in, 3 out]
                  n212 = call "PRI Get Trigger Level.vi"("SlotId"=w509, "DevIdx"=w510) -> ("TriggerLevel"=w500:i32)  [unwired: 1 in, 2 out]
                  n213 = call "PRI Get Frequency Limits.vi"("SlotId"=w509, "DevIdx"=w510) -> ("MaxFreq"=w522:i32, "MinFreq"=w521:i32)  [unwired: 2 in, 2 out]
                  n214 = call "PRI Get Frequency.vi"("SlotId"=w509, "DevIdx"=w510) -> ("Frequency"=w527:i32)  [unwired: 1 in, 2 out]
                  n215 = To Single Precision Float(number=w527) -> (single precision float=w525:sgl)
                  n216 = To Single Precision Float(number=w522) -> (single precision float=w524:sgl)
                  n217 = Divide(x=w503, y=w504) -> (x/y=w501:dbl)
                  n218 = To Single Precision Float(number=w521) -> (single precision float=w523:sgl)
                  n219 = Divide(x=w502, y=w504) -> (x/y=w498:dbl)
                  n220 = for {
                    N: w532 -> [_]
                    tunnel: w531 -> [w541] mode=indexing
                    shift-right: [w544] -> w529
                    shift-left: "" -> [w543]
                    i -> [w542]
                    n221 = call <vilib>:"Trim Whitespace.vi"("string"=w541) -> ("trimmed string"=w540:string)  [unwired: 1 in]
                    n222 = Format Into String(format string="\\t\\t\\s\\strig.\\ssrc.\\s[%d]\\s\\s\\s\\s=\\s\\s'%s'\\n", initial string=w543, w542, w540) -> (resulting string=w544:string)  [unwired: 1 in, 1 out]
                  }
                  n223 = Divide(x=w500, y=w504) -> (x/y=w499:dbl)
                  n224 = call "PRI Decode Trigger Source.vi"("DevIdx"=w510, "SlotId"=w509, "TrigSrc_Idx"=w507) -> ("Freq Enabled"=w535:bool, "TrigLvl Enabled"=w511:bool, "TrigSrc"=w519:string)  [unwired: 1 in, 2 out]
                  n225 = Select(t="", s=w535, f="in") -> (s? t:f=w528:string)
                  n226 = Select(t="", s=w511, f="in") -> (s? t:f=w506:string)
                  n227 = Format Into String(format string="\\t\\tfor TS-Idx = %d\\s\\s\\s\\s\\s\\s:\\s\\sfrequency is %sactive:\\n\\t\\t\\s\\sfrequency\\srange\\s\\s\\s=\\s\\s%.0pHz\\s<= f <=\\s%.0pHz\\n\\t\\t\\s\\scur.\\sfrequency\\s\\s\\s\\s=\\s\\s%.0pHz\\n", initial string="", w507, w528, w523, w524, w525) -> (resulting string=w520:string)  [unwired: 1 in, 1 out]
                  n228 = Format Into String(format string="\\t\\tfor TS-Idx = %d\\s\\s\\s\\s\\s\\s:\\s\\strigger level is %sactive:\\n\\t\\t\\s\\strig.lvl.\\srange\\s\\s\\s=\\s\\s%.3fV\\s<= tl <=\\s%.3fV\\n\\t\\t\\s\\scur. trig.lvl.\\s\\s\\s\\s=\\s\\s%.3fV\\n", initial string="", w507, w506, w501, w498, w499) -> (resulting string=w505:string)  [unwired: 1 in, 1 out]
                  n229 = call <vilib>:"Trim Whitespace.vi"("string"=w519) -> ("trimmed string"=w517:string)  [unwired: 1 in]
                  n230 = String Length(string=w517) -> (length=w515:i32)
                  n231 = String Subset(string="';             ", offset (0)=w515) -> (substring=w518:string)  [unwired: 1 in]
                  n232 = Format Into String(format string="\t\ttrigger sources     =  %d\n%s\t\tcur. trig. source   =  '%s';%sTS-Idx=%d\n\n%s\n%s\n", initial string=w538, w532, w529, w517, w518, w507, w520, w505) -> (resulting string=w537:string)  [unwired: 1 in, 1 out]
                }
                frame 3 {
                  n233 = call "PRI Get Wavelength Index.vi"("SlotId"=w556, "DevIdx"=w557) -> ("Wavelength_Idx"=w547:i32)  [unwired: 1 in, 2 out]
                  n234 = call "PRI Get Intensity.vi"("Wavelength Idx"=w547, "SlotId"=w556, "DevIdx"=w557) -> ("Intensity"=w554:u16)  [unwired: 1 in, 2 out]
                  n235 = To Double Precision Float(number=w554) -> (double precision float=w555:dbl)
                  n236 = Multiply(x=w555, y=0.1) -> (x*y=w551:dbl)
                  n237 = Format Into String(format string="%.1f" ("string"), initial string="", w551) -> (resulting string=w548:string)  [unwired: 1 in, 1 out]
                  n238 = String Length(string=w548) -> (length=w553:i32)
                  n239 = String Subset(string=";              ", offset (0)=w553) -> (substring=w546:string)  [unwired: 1 in]
                  n240 = Format Into String(format string="\t\tintensity           =  %s\\%; %sWL-Idx=%d\n\n", initial string=w559, w548, w546, w547) -> (resulting string=w560:string)  [unwired: 1 in, 1 out]
                }
                frame 4 {
                  w578 = 1e-09 ("x")
                  n241 = call "PRI Get Gating Limits.vi"("SlotId"=w572, "DevIdx"=w573) -> ("MaxOnTime"=w576:i32, "MinOnTime"=w577:i32, "MaxOffTimeFactor"=w570:i32, "MinOffTimeFactor"=w571:i32)  [unwired: 2 in, 2 out]
                  n242 = call "PRI Get Gating Data.vi"("SlotId"=w572, "DevIdx"=w573) -> ("OffTimeFactor"=w567:i32, "OnTime"=w582:i32)  [unwired: 2 in, 2 out]
                  n243 = call "PRI Get Gate High Impedance.vi"("SlotId"=w572, "DevIdx"=w573) -> ("Gate High Impedance"=w592:bool)  [unwired: 1 in, 2 out]
                  n244 = call "PRI Get Gating Enabled.vi"("SlotId"=w572, "DevIdx"=w573) -> ("Gating Enabled"=w583:bool)  [unwired: 1 in, 2 out]
                  n245 = Select(t="en", s=w583, f="dis") -> (s? t:f=w584:string)
                  n246 = Select(t="high (>= 1 kOhm)", s=w592, f="low (~ 50 Ohm)") -> (s? t:f=w585:string)
                  n247 = To Single Precision Float(number=w577) -> (single precision float=w580:sgl)
                  n248 = To Single Precision Float(number=w576) -> (single precision float=w579:sgl)
                  n249 = To Single Precision Float(number=w582) -> (single precision float=w581:sgl)
                  n250 = Multiply(x=w578, y=w580) -> (x*y=w575:dbl)
                  n251 = Multiply(x=w578, y=w579) -> (x*y=w574:dbl)
                  n252 = Multiply(x=w578, y=w581) -> (x*y=w565:dbl)
                  n253 = Increment(x=w567) -> (x+1=w564:i32)
                  n254 = To Single Precision Float(number=w567) -> (single precision float=w569:sgl)
                  n255 = To Single Precision Float(number=w564) -> (single precision float=w566:sgl)
                  n256 = Multiply(x=w565, y=w569) -> (x*y=w568:dbl)
                  n257 = Multiply(x=w565, y=w566) -> (x*y=w562:dbl)
                  n258 = Reciprocal(x=w562) -> (1/x=w563:dbl)
                  n259 = Format Into String(format string="\t\tgating              =  %sabled\n\t\t  gate impedance    =  %s\n\t\t  on-time range     =  %.1ps <= t <= %.1ps\n\t\t  cur. on-time      =  %.1ps\n\t\t  off-t.fact range  =  %d <= tf <= %d\n\t\t  cur. off-time     =  %d * on-time = %.3ps\n\t\t  gate period       =  %.3ps\n\t\t  gate frequency    =  %.3pHz\n", initial string=w588, w584, w585, w575, w574, w565, w571, w570, w567, w568, w562, w563) -> (resulting string=w589:string)  [unwired: 1 in, 1 out]
                }
                frame Default {
                }
              }
            }
          }
          frame 192 {
            w597 = "\t"
            # "FRMS"
            n260 = Concatenate Strings(w597, w597, "backplane (type \"S\")") -> (w595:string)
          }
          frame 200 {
            w600 = "\t"
            # "FRML"
            n261 = Concatenate Strings(w600, w600, "backplane (type \"L\")") -> (w598:string)
          }
          frame 255, Default {
            # "unknown module types"
          }
        }
        n262 = call "COM Get Serial Number.vi"("GetPrimary"=w67, "SlotId"=w62, "DevIdx"=w68) -> ("SerialNumber"=w60:string)  [unwired: 1 in, 2 out]
        n263 = call "COM Decode Module Type.vi"("ModuleType"=w69) -> ("ModulType"=w61:string)  [unwired: 1 in, 2 out]
        n264 = Format Into String(format string="%s\\n\\t%03d :\\t%s\\n\\t\\tserial number\\s\\s\\s\\s\\s\\s\\s:\\s\\s\\'%s\\'\\n%s\\n", initial string="", w65, w62, w61, w60, w59) -> (resulting string=w63:string)  [unwired: 1 in, 1 out]
      }
      frame -1, Default {
        n265 = Format Into String(format string="%s\\n\\t%03d :\\t%s\\n", initial string="", w605, w603, "unknown Module type") -> (resulting string=w604:string)  [unwired: 1 in, 1 out]
      }
      frame -9008 {
        n266 = Format Into String(format string="%s\\n\\t%03d :\\t%s\\n", initial string="", w611, w609, "n/a") -> (resulting string=w610:string)  [unwired: 1 in, 1 out]
      }
      frame -9009 {
        n267 = Format Into String(format string="%s\\n\\t%03d :\\t%s\\n", initial string="", w617, w615, "empty slot") -> (resulting string=w616:string)  [unwired: 1 in, 1 out]
      }
    }
    n268 = feedback-in #1(w58) -> ()
  }
  "cModulesDisplay" <- w29
  n269 = control-ref of="This VI"() -> (w8:refnum<vi>)
  n270 = property class="VI"(reference=w8) -> ("Name"=w10:string)  [unwired: 1 in, 2 out]
  n271 = call "FWR Create Support Request Text.vi"("DevIdx"="iDevIdx", "Preamble"="", "CallingSW"=w10, "error in (no error)"=w13, "Options"=0) -> ("SupportRequestText"=w4:string, "error out"=w3:errorcluster)  [unwired: 1 out]
  n272 = case shown="True" "CreateSupportRequest" {
    tunnel: w4 -> [_ w627]
    tunnel: w3 -> [w620 w626]
    tunnel: [w620 w621] -> w1
    frame False {
    }
    frame True {
      n273 = Get Date/Time In Seconds() -> (seconds since 1Jan1904=w636:timestamp)
      n274 = Format Date/Time String(time format string (%c)="_%Y%m%d_%H%M%S.txt", seconds (now)=w636) -> (date/time string=w632:string)  [unwired: 1 in]
      n275 = local read "cSerialNumber"() -> (w633:string)
      n276 = Current VI's Path() -> (path=w625:path)
      n277 = Strip Path(path=w625) -> (stripped path=w624:path)  [unwired: 1 out]
      n278 = Path To String(path=w624) -> (string=w630:string)
      n279 = Concatenate Strings(w630, "\\", "ServiceRequest_SN", w633, w632) -> (w629:string)
      n280 = String To Path(string=w629) -> (path=w628:path)
      n281 = Write to Text File(file (use dialog)=w628, text=w627, error in=w626) -> (refnum out=w622:refnum<file>, error out=w623:errorcluster)  [unwired: 1 in, 1 out]
      n282 = Close File(refnum=w622, error in=w623) -> (error out=w621:errorcluster)  [unwired: 1 out]
    }
  }
  n283 = call "FWR Free Module Map.vi"("error in (no error)"=w1, "DevIdx"="iDevIdx") -> ("error out"=w31:errorcluster)  [unwired: 1 out]
  n284 = Search and Replace String(input string=w4, search string="\r\n", replace string="\n") -> (result string=→"cSupportRequestText":string)  [unwired: 5 in, 3 out]
  n285 = call "USB Close Device.vi"("error in (no error)"=w31, "DevIdx"="iDevIdx") -> ("error out"=→"error out":errorcluster)
